vi "SetRingItemString.vi"(8 "error in (no error)":errorcluster, 9 "Strings []":string[](array[string]), 10 "TargetCtlLabel.Text":string="SourceSelect", 11 "AllControlReference":refnum<vi>[](array[refnum])) -> (0 "error out":errorcluster)   [LabVIEW 2013, in "Initialize.lvclass"]
uses:
  Initialize.lvclass
panel:
  in  "InstrumentSelect":u16(ring) items=["儀器1"]
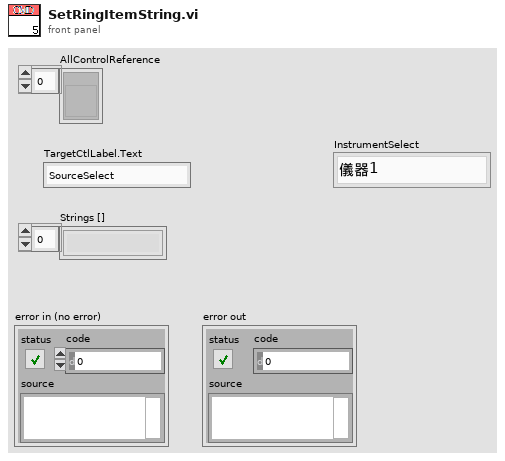
[diagram p1: front panel]
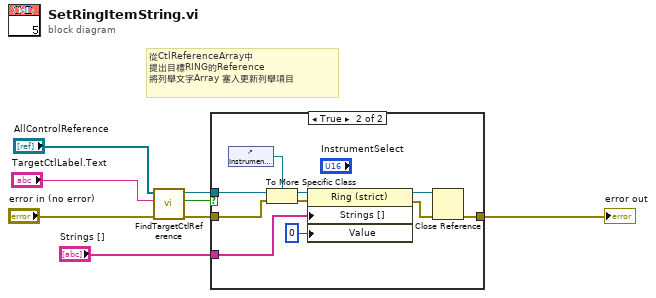
[diagram p0: block diagram]
diagram:
  # "從CtlReferenceArray中\n提出目標RING的Reference\n將列舉文字Array 塞入更新列舉項目"
  n1 = call "FindTargetCtlReference.vi"("error in (no error)"="error in (no error)", "TargetCtlLabel.Text"="TargetCtlLabel.Text", "AllControlReference"="AllControlReference") -> ("error out"=w5:errorcluster, "Find?"=w4:bool, "TargetCtlRefnum"=w6:refnum<vi>)  [unwired: 6 in]
  n2 = case shown="True" w4 {
    tunnel: w5 -> [w9 w18]
    tunnel: w6 -> [_ w19]
    tunnel: [w9 w14] -> w7
    tunnel: "Strings []" -> [_ w12]
    frame False {
    }
    frame True {
      n3 = control-ref of="InstrumentSelect"() -> (w11:refnum<vi>)
      n4 = To More Specific Class(target class=w11, reference=w19, error in=w18) -> (specific class reference=w17:refnum<vi>, error out=w16:errorcluster)
      n5 = property class="Ring (strict)"(reference=w17, error in=w16, "Strings []"=w12, "Value"=u16 0) -> (reference out=w13:refnum<vi>, error out=w15:errorcluster)
      n6 = Close Reference(reference=w13, error in (no error)=w15) -> (error out=w14:errorcluster)
    }
  }
  "error out" <- w7
